vi "SERIAL_DecodeASCII.vi"(2 "navX Data":u8[](array[numeric]), 3 "Buffer":string) -> (0 "navX Data":u8[](array[numeric]), 1 "Valid?":bool)   [LabVIEW 2014, in "navX-MXP IMU.lvlib"]
uses:
  navX-MXP IMU.lvlib
  COMMON/TypeDefs/Value TypeDefs/navX Device Registers.ctl
  COMMON/TypeDefs/Value TypeDefs/navX NAVX_CAL_STATUS.ctl
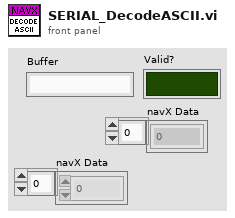
[diagram p1: front panel]
types:
  T1 = typedef "navX-MXP IMU.lvlib/navX Device Registers.ctl" = u8
  T2 = typedef "navX-MXP IMU.lvlib/navX NAVX_CAL_STATUS.ctl" = u8
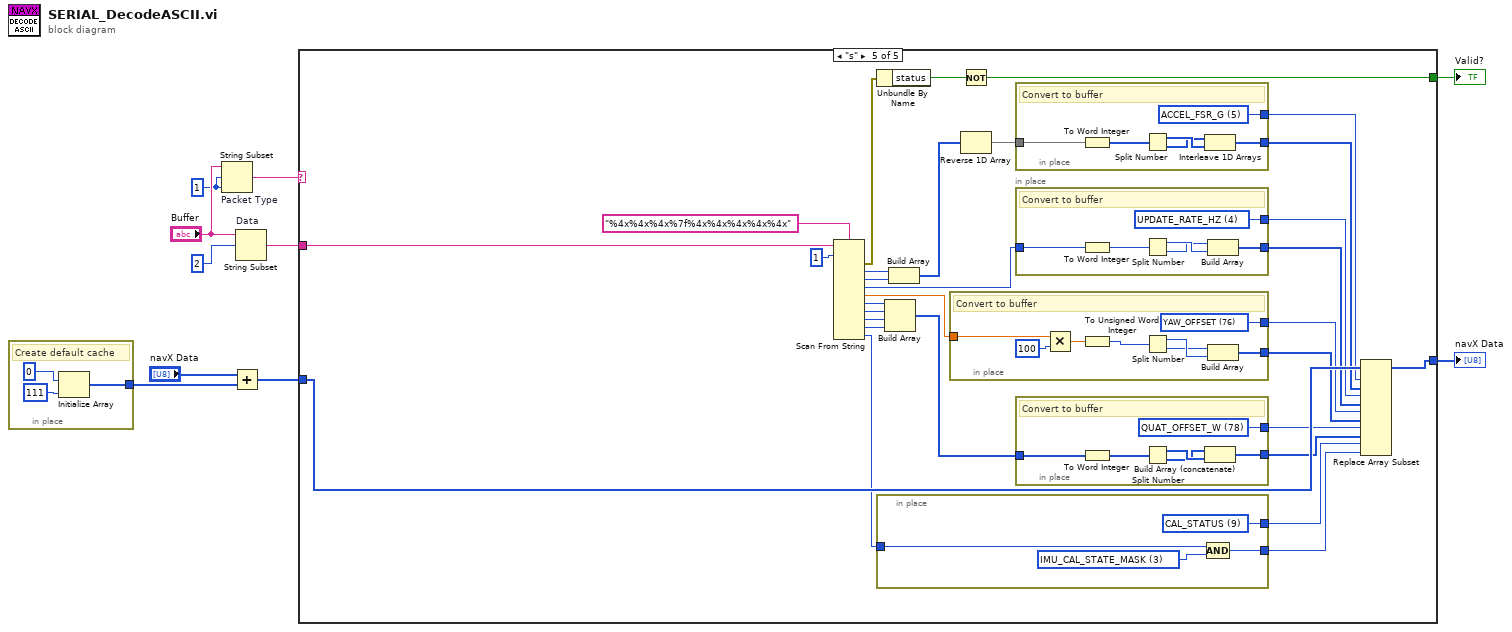
[diagram p0: block diagram]
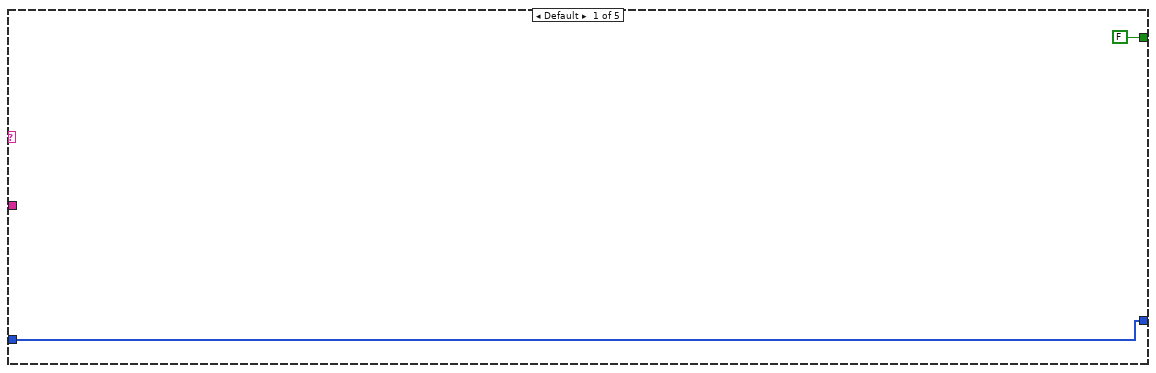
[diagram p2: hidden frame]
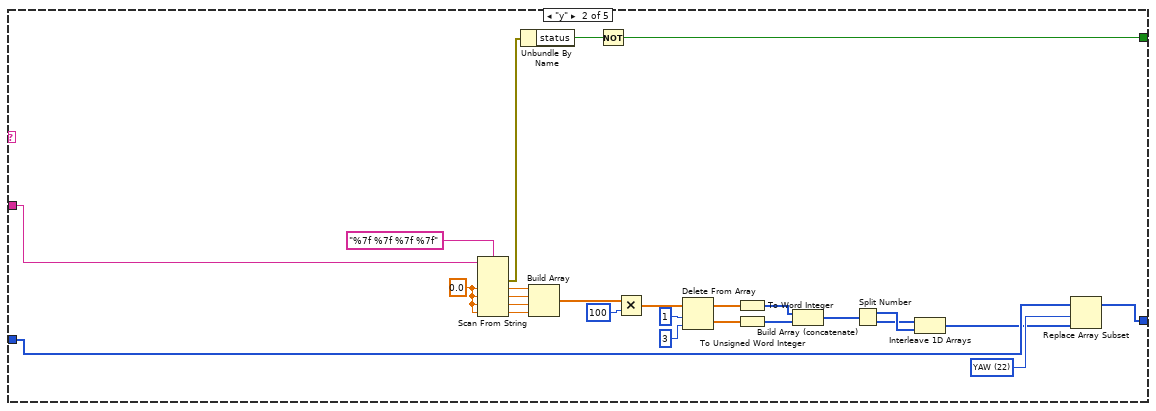
[diagram p3: hidden frame]
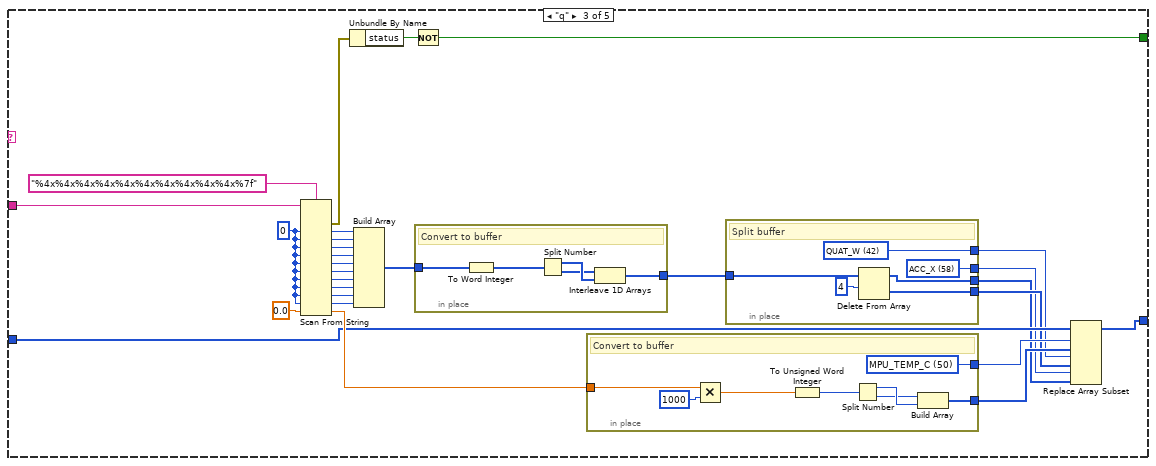
[diagram p4: hidden frame]
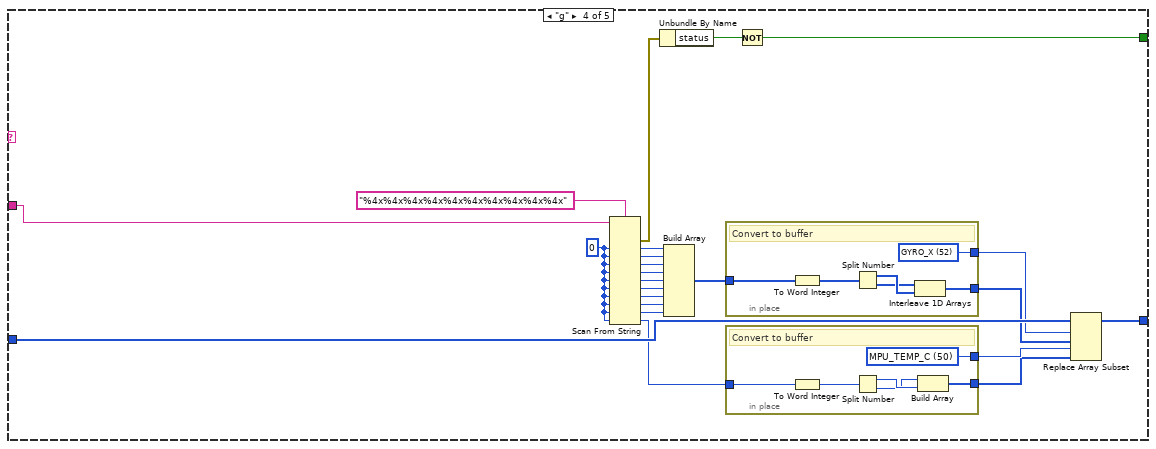
[diagram p5: hidden frame]
diagram:
  w8 = 1 ("offset (0)")
  n1 = in-place {
    in-place-border: [w11] -> w3
    # "Create default cache"
    n2 = Initialize Array(u8 0 ("Received Data"), u8 111 ("hex")) -> (w11:u8[])
  }
  n3 = String Subset "Packet Type"(string="Buffer", offset (0)=w8, length (rest)=w8) -> (substring=w7:string)
  n4 = Add(x="navX Data", y=w3) -> (x+y=w2:u8[])
  n5 = String Subset "Data"(string="Buffer", offset (0)=2) -> (substring=w1:string)  [unwired: 1 in]
  n6 = case shown="\"s\"" w7 {
    tunnel: w1 -> [_ w40 w65 w89 w124]
    tunnel: w2 -> [w15 w32 w50 w100 w147]
    tunnel: [w15 w30 w49 w97 w148] -> w6
    tunnel: [FALSE w16 w51 w94 w149] -> w5
    frame Default {
    }
    frame "y" {
      w31 = T1 22 items=["WHOAMI"=0, "HW_REV"=1, "FW_VER_MAJOR"=2, "FW_VER_MINOR"=3, "UPDATE_RATE_HZ"=4, "ACCEL_FSR_G"=5, "GYRO_FSR_DPS"=6, "OP_STATUS"=8, "CAL_STATUS"=9, "SELFTEST_STATUS"=10, "CAPABILITY_FLAGS_L"=11, "CAPABILITY_FLAGS_H"=12, "SENSOR_STATUS"=16, "TIMESTAMP"=18, "YAW"=22, "PITCH"=24, "ROLL"=26, "HEADING"=28, "FUSED_HEADING"=30, "ALTITUDE_I"=32, "ALTITUDE_D"=34, "LINERA_ACC_X"=36, "LINERA_ACC_Y"=38, "LINERA_ACC_Z"=40, "QUAT_W"=42, "QUAT_X"=44, "QUAT_Y"=46, "QUAT_Z"=48, "MPU_TEMP_C"=50, "GYRO_X"=52, "GYRO_Y"=54, "GYRO_Z"=56, "ACC_X"=58, "ACC_Y"=60, "ACC_Z"=62, "MAG_X"=64, "MAG_Y"=66, "MAG_Z"=68, "PRESSURE_I"=70, "PRESSURE_D"=72, "PRESSURE_TEMP"=74, "YAW_OFFSET"=76, "QUAT_OFFSET_W"=78, "QUAT_OFFSET_X"=80, "QUAT_OFFSET_Y"=82, "QUAT_OFFSET_Z"=84, "INTEGRATION_CONTROL"=86, "VELOCITY_X"=88, "VELOCITY_Y"=92, "VELOCITY_Z"=96, "DISPLACMENT_X"=100, "DISPLACMENT_Y"=104, "DISPLACEMENT_Z"=108] ("Device Register")
      w39 = 0.0 ("default value 1")
      n7 = Scan From String(format string="%7f %7f %7f %7f", input string=w40, default 1=w39, default 2=w39, default 3=w39, default 4=w39) -> (error out=w18:errorcluster, output 1=w38:dbl, output 2=w35:dbl, output 3=w36:dbl, output 4=w37:dbl)  [unwired: 2 in, 2 out]
      n8 = Unbundle By Name(w18) -> ("status"=w17:bool)
      n9 = Build Array(w38, w35, w36, w37) -> (w34:dbl[])
      n10 = Not(x=w17) -> (.not. x?=w16:bool)
      n11 = Multiply(x=w34, y=u16 100) -> (x*y=w20:dbl[])
      n12 = Delete From Array(array=w20, length=1, index=3) -> (deleted portion=w25:dbl[], array with subset deleted=w24:dbl[])
      n13 = To Word Integer(number=w24) -> (16bit integer=w23:i16[])
      n14 = To Unsigned Word Integer(number=w25) -> (unsigned 16bit integer=w22:u16[])
      n15 = Build Array (concatenate)(w23, w22) -> (w21:u16[])
      n16 = Split Number(x=w21) -> (hi(x)=w29:u8[], lo(x)=w28:u8[])
      n17 = Interleave 1D Arrays(w28, w29) -> (w19:u8[])
      n18 = Replace Array Subset(array=w32, new element=w19, index=w31) -> (w30:u8[])
    }
    frame "q" {
      w66 = u32 0 ("default value 1")
      n19 = Scan From String(format string="%4x%4x%4x%4x%4x%4x%4x%4x%4x%4x%7f", input string=w65, default 1=w66, default 2=w66, default 3=w66, default 4=w66, default 5=w66, default 6=w66, default 7=w66, default 8=w66, default 9=w66, default 10=w66, default 11=0.0 ("default value 11")) -> (error out=w67:errorcluster, output 1=w62:u32, output 2=w61:u32, output 3=w60:u32, output 4=w59:u32, output 5=w58:u32, output 6=w57:u32, output 7=w56:u32, output 8=w55:u32, output 9=w54:u32, output 10=w53:u32, output 11=w52:dbl)  [unwired: 2 in, 2 out]
      n20 = Unbundle By Name(w67) -> ("status"=w68:bool)
      n21 = Build Array(w62, w61, w60, w59, w58, w57, w56, w55, w54, w53) -> (w63:u32[])
      n22 = Not(x=w68) -> (.not. x?=w51:bool)
      n23 = in-place {
        in-place-border: w63 -> [w88]
        in-place-border: [w84] -> w46
        # "Convert to buffer"
        n24 = To Word Integer(number=w88) -> (16bit integer=w85:i16[])
        n25 = Split Number(x=w85) -> (hi(x)=w87:u8[], lo(x)=w86:u8[])
        n26 = Interleave 1D Arrays(w86, w87) -> (w84:u8[])
      }
      n27 = in-place {
        in-place-border: w52 -> [w80]
        in-place-border: [w77] -> w47
        in-place-border: [w76] -> w48
        w76 = T1 50 items=["WHOAMI"=0, "HW_REV"=1, "FW_VER_MAJOR"=2, "FW_VER_MINOR"=3, "UPDATE_RATE_HZ"=4, "ACCEL_FSR_G"=5, "GYRO_FSR_DPS"=6, "OP_STATUS"=8, "CAL_STATUS"=9, "SELFTEST_STATUS"=10, "CAPABILITY_FLAGS_L"=11, "CAPABILITY_FLAGS_H"=12, "SENSOR_STATUS"=16, "TIMESTAMP"=18, "YAW"=22, "PITCH"=24, "ROLL"=26, "HEADING"=28, "FUSED_HEADING"=30, "ALTITUDE_I"=32, "ALTITUDE_D"=34, "LINERA_ACC_X"=36, "LINERA_ACC_Y"=38, "LINERA_ACC_Z"=40, "QUAT_W"=42, "QUAT_X"=44, "QUAT_Y"=46, "QUAT_Z"=48, "MPU_TEMP_C"=50, "GYRO_X"=52, "GYRO_Y"=54, "GYRO_Z"=56, "ACC_X"=58, "ACC_Y"=60, "ACC_Z"=62, "MAG_X"=64, "MAG_Y"=66, "MAG_Z"=68, "PRESSURE_I"=70, "PRESSURE_D"=72, "PRESSURE_TEMP"=74, "YAW_OFFSET"=76, "QUAT_OFFSET_W"=78, "QUAT_OFFSET_X"=80, "QUAT_OFFSET_Y"=82, "QUAT_OFFSET_Z"=84, "INTEGRATION_CONTROL"=86, "VELOCITY_X"=88, "VELOCITY_Y"=92, "VELOCITY_Z"=96, "DISPLACMENT_X"=100, "DISPLACMENT_Y"=104, "DISPLACEMENT_Z"=108] ("Device Register")
        # "Convert to buffer"
        n28 = Multiply(x=w80, y=u16 1000) -> (x*y=w79:dbl)
        n29 = To Unsigned Word Integer(number=w79) -> (unsigned 16bit integer=w78:u16)
        n30 = Split Number(x=w78) -> (hi(x)=w82:u8, lo(x)=w81:u8)
        n31 = Build Array(w81, w82) -> (w77:u8[])
      }
      n32 = in-place {
        in-place-border: w46 -> [w75]
        in-place-border: [w73] -> w45
        in-place-border: [w72] -> w44
        in-place-border: [w71] -> w43
        in-place-border: [w70] -> w42
        w70 = T1 58 items=["WHOAMI"=0, "HW_REV"=1, "FW_VER_MAJOR"=2, "FW_VER_MINOR"=3, "UPDATE_RATE_HZ"=4, "ACCEL_FSR_G"=5, "GYRO_FSR_DPS"=6, "OP_STATUS"=8, "CAL_STATUS"=9, "SELFTEST_STATUS"=10, "CAPABILITY_FLAGS_L"=11, "CAPABILITY_FLAGS_H"=12, "SENSOR_STATUS"=16, "TIMESTAMP"=18, "YAW"=22, "PITCH"=24, "ROLL"=26, "HEADING"=28, "FUSED_HEADING"=30, "ALTITUDE_I"=32, "ALTITUDE_D"=34, "LINERA_ACC_X"=36, "LINERA_ACC_Y"=38, "LINERA_ACC_Z"=40, "QUAT_W"=42, "QUAT_X"=44, "QUAT_Y"=46, "QUAT_Z"=48, "MPU_TEMP_C"=50, "GYRO_X"=52, "GYRO_Y"=54, "GYRO_Z"=56, "ACC_X"=58, "ACC_Y"=60, "ACC_Z"=62, "MAG_X"=64, "MAG_Y"=66, "MAG_Z"=68, "PRESSURE_I"=70, "PRESSURE_D"=72, "PRESSURE_TEMP"=74, "YAW_OFFSET"=76, "QUAT_OFFSET_W"=78, "QUAT_OFFSET_X"=80, "QUAT_OFFSET_Y"=82, "QUAT_OFFSET_Z"=84, "INTEGRATION_CONTROL"=86, "VELOCITY_X"=88, "VELOCITY_Y"=92, "VELOCITY_Z"=96, "DISPLACMENT_X"=100, "DISPLACMENT_Y"=104, "DISPLACEMENT_Z"=108] ("Device Register")
        w72 = T1 42 items=["WHOAMI"=0, "HW_REV"=1, "FW_VER_MAJOR"=2, "FW_VER_MINOR"=3, "UPDATE_RATE_HZ"=4, "ACCEL_FSR_G"=5, "GYRO_FSR_DPS"=6, "OP_STATUS"=8, "CAL_STATUS"=9, "SELFTEST_STATUS"=10, "CAPABILITY_FLAGS_L"=11, "CAPABILITY_FLAGS_H"=12, "SENSOR_STATUS"=16, "TIMESTAMP"=18, "YAW"=22, "PITCH"=24, "ROLL"=26, "HEADING"=28, "FUSED_HEADING"=30, "ALTITUDE_I"=32, "ALTITUDE_D"=34, "LINERA_ACC_X"=36, "LINERA_ACC_Y"=38, "LINERA_ACC_Z"=40, "QUAT_W"=42, "QUAT_X"=44, "QUAT_Y"=46, "QUAT_Z"=48, "MPU_TEMP_C"=50, "GYRO_X"=52, "GYRO_Y"=54, "GYRO_Z"=56, "ACC_X"=58, "ACC_Y"=60, "ACC_Z"=62, "MAG_X"=64, "MAG_Y"=66, "MAG_Z"=68, "PRESSURE_I"=70, "PRESSURE_D"=72, "PRESSURE_TEMP"=74, "YAW_OFFSET"=76, "QUAT_OFFSET_W"=78, "QUAT_OFFSET_X"=80, "QUAT_OFFSET_Y"=82, "QUAT_OFFSET_Z"=84, "INTEGRATION_CONTROL"=86, "VELOCITY_X"=88, "VELOCITY_Y"=92, "VELOCITY_Z"=96, "DISPLACMENT_X"=100, "DISPLACMENT_Y"=104, "DISPLACEMENT_Z"=108] ("Device Register")
        # "Split buffer"
        n33 = Delete From Array(array=w75, length=4) -> (deleted portion=w73:u8[], array with subset deleted=w71:u8[])  [unwired: 1 in]
      }
      n34 = Replace Array Subset(array=w50, new element #1=w47, index #1=w48, new element #2=w45, index #2=w44, new element #3=w43, index #3=w42) -> (w49:u8[])
    }
    frame "g" {
      w90 = u32 0 ("default value 1")
      n35 = Scan From String(format string="%4x%4x%4x%4x%4x%4x%4x%4x%4x%4x", input string=w89, default 1=w90, default 2=w90, default 3=w90, default 4=w90, default 5=w90, default 6=w90, default 7=w90, default 8=w90, default 9=w90, default 10=w90) -> (error out=w95:errorcluster, output 1=w110:u32, output 2=w109:u32, output 3=w108:u32, output 4=w106:u32, output 5=w105:u32, output 6=w104:u32, output 7=w103:u32, output 8=w102:u32, output 9=w101:u32, output 10=w93:u32)  [unwired: 2 in, 2 out]
      n36 = Unbundle By Name(w95) -> ("status"=w96:bool)
      n37 = Build Array(w110, w109, w108, w106, w105, w104, w103, w102, w101) -> (w107:u32[])
      n38 = in-place {
        in-place-border: w107 -> [w123]
        in-place-border: [w119] -> w99
        in-place-border: [w118] -> w98
        w118 = T1 52 items=["WHOAMI"=0, "HW_REV"=1, "FW_VER_MAJOR"=2, "FW_VER_MINOR"=3, "UPDATE_RATE_HZ"=4, "ACCEL_FSR_G"=5, "GYRO_FSR_DPS"=6, "OP_STATUS"=8, "CAL_STATUS"=9, "SELFTEST_STATUS"=10, "CAPABILITY_FLAGS_L"=11, "CAPABILITY_FLAGS_H"=12, "SENSOR_STATUS"=16, "TIMESTAMP"=18, "YAW"=22, "PITCH"=24, "ROLL"=26, "HEADING"=28, "FUSED_HEADING"=30, "ALTITUDE_I"=32, "ALTITUDE_D"=34, "LINERA_ACC_X"=36, "LINERA_ACC_Y"=38, "LINERA_ACC_Z"=40, "QUAT_W"=42, "QUAT_X"=44, "QUAT_Y"=46, "QUAT_Z"=48, "MPU_TEMP_C"=50, "GYRO_X"=52, "GYRO_Y"=54, "GYRO_Z"=56, "ACC_X"=58, "ACC_Y"=60, "ACC_Z"=62, "MAG_X"=64, "MAG_Y"=66, "MAG_Z"=68, "PRESSURE_I"=70, "PRESSURE_D"=72, "PRESSURE_TEMP"=74, "YAW_OFFSET"=76, "QUAT_OFFSET_W"=78, "QUAT_OFFSET_X"=80, "QUAT_OFFSET_Y"=82, "QUAT_OFFSET_Z"=84, "INTEGRATION_CONTROL"=86, "VELOCITY_X"=88, "VELOCITY_Y"=92, "VELOCITY_Z"=96, "DISPLACMENT_X"=100, "DISPLACMENT_Y"=104, "DISPLACEMENT_Z"=108] ("Device Register")
        # "Convert to buffer"
        n39 = To Word Integer(number=w123) -> (16bit integer=w120:i16[])
        n40 = Split Number(x=w120) -> (hi(x)=w122:u8[], lo(x)=w121:u8[])
        n41 = Interleave 1D Arrays(w121, w122) -> (w119:u8[])
      }
      n42 = in-place {
        in-place-border: w93 -> [w113]
        in-place-border: [w115] -> w92
        in-place-border: [w114] -> w91
        w115 = T1 50 items=["WHOAMI"=0, "HW_REV"=1, "FW_VER_MAJOR"=2, "FW_VER_MINOR"=3, "UPDATE_RATE_HZ"=4, "ACCEL_FSR_G"=5, "GYRO_FSR_DPS"=6, "OP_STATUS"=8, "CAL_STATUS"=9, "SELFTEST_STATUS"=10, "CAPABILITY_FLAGS_L"=11, "CAPABILITY_FLAGS_H"=12, "SENSOR_STATUS"=16, "TIMESTAMP"=18, "YAW"=22, "PITCH"=24, "ROLL"=26, "HEADING"=28, "FUSED_HEADING"=30, "ALTITUDE_I"=32, "ALTITUDE_D"=34, "LINERA_ACC_X"=36, "LINERA_ACC_Y"=38, "LINERA_ACC_Z"=40, "QUAT_W"=42, "QUAT_X"=44, "QUAT_Y"=46, "QUAT_Z"=48, "MPU_TEMP_C"=50, "GYRO_X"=52, "GYRO_Y"=54, "GYRO_Z"=56, "ACC_X"=58, "ACC_Y"=60, "ACC_Z"=62, "MAG_X"=64, "MAG_Y"=66, "MAG_Z"=68, "PRESSURE_I"=70, "PRESSURE_D"=72, "PRESSURE_TEMP"=74, "YAW_OFFSET"=76, "QUAT_OFFSET_W"=78, "QUAT_OFFSET_X"=80, "QUAT_OFFSET_Y"=82, "QUAT_OFFSET_Z"=84, "INTEGRATION_CONTROL"=86, "VELOCITY_X"=88, "VELOCITY_Y"=92, "VELOCITY_Z"=96, "DISPLACMENT_X"=100, "DISPLACMENT_Y"=104, "DISPLACEMENT_Z"=108] ("Device Register")
        # "Convert to buffer"
        n43 = To Word Integer(number=w113) -> (16bit integer=w112:i16)
        n44 = Split Number(x=w112) -> (hi(x)=w117:u8, lo(x)=w116:u8)
        n45 = Build Array(w116, w117) -> (w114:u8[])
      }
      n46 = Not(x=w96) -> (.not. x?=w94:bool)
      n47 = Replace Array Subset(array=w100, new element #1=w99, index #1=w98, new element #2=w91, index #2=w92) -> (w97:u8[])
    }
    frame "s" {
      n48 = Scan From String(format string="%4x%4x%4x%7f%4x%4x%4x%4x%4x", input string=w124, initial scan location=u32 1) -> (error out=w150:errorcluster, output 1=w146:u32, output 2=w145:u32, output 3=w140:u32, output 4=w137:dbl, output 5=w134:u32, output 6=w133:u32, output 7=w132:u32, output 8=w131:u32, output 9=w127:u32)  [unwired: 10 in, 2 out]
      n49 = Unbundle By Name(w150) -> ("status"=w151:bool)
      n50 = in-place {
        in-place-border: w127 -> [w156]
        in-place-border: [w155] -> w126
        in-place-border: [w154] -> w125
        w155 = T1 9 items=["WHOAMI"=0, "HW_REV"=1, "FW_VER_MAJOR"=2, "FW_VER_MINOR"=3, "UPDATE_RATE_HZ"=4, "ACCEL_FSR_G"=5, "GYRO_FSR_DPS"=6, "OP_STATUS"=8, "CAL_STATUS"=9, "SELFTEST_STATUS"=10, "CAPABILITY_FLAGS_L"=11, "CAPABILITY_FLAGS_H"=12, "SENSOR_STATUS"=16, "TIMESTAMP"=18, "YAW"=22, "PITCH"=24, "ROLL"=26, "HEADING"=28, "FUSED_HEADING"=30, "ALTITUDE_I"=32, "ALTITUDE_D"=34, "LINERA_ACC_X"=36, "LINERA_ACC_Y"=38, "LINERA_ACC_Z"=40, "QUAT_W"=42, "QUAT_X"=44, "QUAT_Y"=46, "QUAT_Z"=48, "MPU_TEMP_C"=50, "GYRO_X"=52, "GYRO_Y"=54, "GYRO_Z"=56, "ACC_X"=58, "ACC_Y"=60, "ACC_Z"=62, "MAG_X"=64, "MAG_Y"=66, "MAG_Z"=68, "PRESSURE_I"=70, "PRESSURE_D"=72, "PRESSURE_TEMP"=74, "YAW_OFFSET"=76, "QUAT_OFFSET_W"=78, "QUAT_OFFSET_X"=80, "QUAT_OFFSET_Y"=82, "QUAT_OFFSET_Z"=84, "INTEGRATION_CONTROL"=86, "VELOCITY_X"=88, "VELOCITY_Y"=92, "VELOCITY_Z"=96, "DISPLACMENT_X"=100, "DISPLACMENT_Y"=104, "DISPLACEMENT_Z"=108] ("Device Register")
        w157 = T2 3 items=["IMU_CAL_STATE_MASK"=3, "IMU_CAL_INPROGRESS"=0, "IMU_CAL_ACCUMULATE"=1, "IMU_CAL_COMPLETE"=2, "MAG_CAL_COMPLETE"=4, "BARO_CAL_COMPLETE"=8] ("NAVX_CAL_STATUS")
        n51 = Compound Arithmetic op=AND(w156, w157) -> (w154:u32)
      }
      n52 = Build Array(w134, w133, w132, w131) -> (w130:u32[])
      n53 = Build Array(w146, w145) -> (w144:u32[])
      n54 = in-place {
        in-place-border: w137 -> [w168]
        in-place-border: [w165] -> w135
        in-place-border: [w164] -> w136
        w164 = T1 76 items=["WHOAMI"=0, "HW_REV"=1, "FW_VER_MAJOR"=2, "FW_VER_MINOR"=3, "UPDATE_RATE_HZ"=4, "ACCEL_FSR_G"=5, "GYRO_FSR_DPS"=6, "OP_STATUS"=8, "CAL_STATUS"=9, "SELFTEST_STATUS"=10, "CAPABILITY_FLAGS_L"=11, "CAPABILITY_FLAGS_H"=12, "SENSOR_STATUS"=16, "TIMESTAMP"=18, "YAW"=22, "PITCH"=24, "ROLL"=26, "HEADING"=28, "FUSED_HEADING"=30, "ALTITUDE_I"=32, "ALTITUDE_D"=34, "LINERA_ACC_X"=36, "LINERA_ACC_Y"=38, "LINERA_ACC_Z"=40, "QUAT_W"=42, "QUAT_X"=44, "QUAT_Y"=46, "QUAT_Z"=48, "MPU_TEMP_C"=50, "GYRO_X"=52, "GYRO_Y"=54, "GYRO_Z"=56, "ACC_X"=58, "ACC_Y"=60, "ACC_Z"=62, "MAG_X"=64, "MAG_Y"=66, "MAG_Z"=68, "PRESSURE_I"=70, "PRESSURE_D"=72, "PRESSURE_TEMP"=74, "YAW_OFFSET"=76, "QUAT_OFFSET_W"=78, "QUAT_OFFSET_X"=80, "QUAT_OFFSET_Y"=82, "QUAT_OFFSET_Z"=84, "INTEGRATION_CONTROL"=86, "VELOCITY_X"=88, "VELOCITY_Y"=92, "VELOCITY_Z"=96, "DISPLACMENT_X"=100, "DISPLACMENT_Y"=104, "DISPLACEMENT_Z"=108] ("Device Register")
        # "Convert to buffer"
        n55 = Multiply(x=w168, y=u16 100) -> (x*y=w167:dbl)
        n56 = To Unsigned Word Integer(number=w167) -> (unsigned 16bit integer=w166:u16)
        n57 = Split Number(x=w166) -> (hi(x)=w170:u8, lo(x)=w169:u8)
        n58 = Build Array(w169, w170) -> (w165:u8[])
      }
      n59 = Not(x=w151) -> (.not. x?=w149:bool)
      n60 = Reverse 1D Array(array=w144) -> (reversed array=w143:u32[])
      n61 = in-place {
        in-place-border: w143 -> [w183]
        in-place-border: [w179] -> w141
        in-place-border: [w178] -> w142
        w178 = T1 5 items=["WHOAMI"=0, "HW_REV"=1, "FW_VER_MAJOR"=2, "FW_VER_MINOR"=3, "UPDATE_RATE_HZ"=4, "ACCEL_FSR_G"=5, "GYRO_FSR_DPS"=6, "OP_STATUS"=8, "CAL_STATUS"=9, "SELFTEST_STATUS"=10, "CAPABILITY_FLAGS_L"=11, "CAPABILITY_FLAGS_H"=12, "SENSOR_STATUS"=16, "TIMESTAMP"=18, "YAW"=22, "PITCH"=24, "ROLL"=26, "HEADING"=28, "FUSED_HEADING"=30, "ALTITUDE_I"=32, "ALTITUDE_D"=34, "LINERA_ACC_X"=36, "LINERA_ACC_Y"=38, "LINERA_ACC_Z"=40, "QUAT_W"=42, "QUAT_X"=44, "QUAT_Y"=46, "QUAT_Z"=48, "MPU_TEMP_C"=50, "GYRO_X"=52, "GYRO_Y"=54, "GYRO_Z"=56, "ACC_X"=58, "ACC_Y"=60, "ACC_Z"=62, "MAG_X"=64, "MAG_Y"=66, "MAG_Z"=68, "PRESSURE_I"=70, "PRESSURE_D"=72, "PRESSURE_TEMP"=74, "YAW_OFFSET"=76, "QUAT_OFFSET_W"=78, "QUAT_OFFSET_X"=80, "QUAT_OFFSET_Y"=82, "QUAT_OFFSET_Z"=84, "INTEGRATION_CONTROL"=86, "VELOCITY_X"=88, "VELOCITY_Y"=92, "VELOCITY_Z"=96, "DISPLACMENT_X"=100, "DISPLACMENT_Y"=104, "DISPLACEMENT_Z"=108] ("Device Register")
        # "Convert to buffer"
        n62 = To Word Integer(number=w183) -> (16bit integer=w180:i16[])
        n63 = Split Number(x=w180) -> (hi(x)=w182:u8[], lo(x)=w181:u8[])
        n64 = Interleave 1D Arrays(w181, w182) -> (w179:u8[])
      }
      n65 = in-place {
        in-place-border: w140 -> [w177]
        in-place-border: [w173] -> w138
        in-place-border: [w172] -> w139
        w172 = T1 4 items=["WHOAMI"=0, "HW_REV"=1, "FW_VER_MAJOR"=2, "FW_VER_MINOR"=3, "UPDATE_RATE_HZ"=4, "ACCEL_FSR_G"=5, "GYRO_FSR_DPS"=6, "OP_STATUS"=8, "CAL_STATUS"=9, "SELFTEST_STATUS"=10, "CAPABILITY_FLAGS_L"=11, "CAPABILITY_FLAGS_H"=12, "SENSOR_STATUS"=16, "TIMESTAMP"=18, "YAW"=22, "PITCH"=24, "ROLL"=26, "HEADING"=28, "FUSED_HEADING"=30, "ALTITUDE_I"=32, "ALTITUDE_D"=34, "LINERA_ACC_X"=36, "LINERA_ACC_Y"=38, "LINERA_ACC_Z"=40, "QUAT_W"=42, "QUAT_X"=44, "QUAT_Y"=46, "QUAT_Z"=48, "MPU_TEMP_C"=50, "GYRO_X"=52, "GYRO_Y"=54, "GYRO_Z"=56, "ACC_X"=58, "ACC_Y"=60, "ACC_Z"=62, "MAG_X"=64, "MAG_Y"=66, "MAG_Z"=68, "PRESSURE_I"=70, "PRESSURE_D"=72, "PRESSURE_TEMP"=74, "YAW_OFFSET"=76, "QUAT_OFFSET_W"=78, "QUAT_OFFSET_X"=80, "QUAT_OFFSET_Y"=82, "QUAT_OFFSET_Z"=84, "INTEGRATION_CONTROL"=86, "VELOCITY_X"=88, "VELOCITY_Y"=92, "VELOCITY_Z"=96, "DISPLACMENT_X"=100, "DISPLACMENT_Y"=104, "DISPLACEMENT_Z"=108] ("Device Register")
        # "Convert to buffer"
        n66 = To Word Integer(number=w177) -> (16bit integer=w174:i16)
        n67 = Split Number(x=w174) -> (hi(x)=w176:u8, lo(x)=w175:u8)
        n68 = Build Array(w175, w176) -> (w173:u8[])
      }
      n69 = in-place {
        in-place-border: w130 -> [w163]
        in-place-border: [w159] -> w128
        in-place-border: [w158] -> w129
        w158 = T1 78 items=["WHOAMI"=0, "HW_REV"=1, "FW_VER_MAJOR"=2, "FW_VER_MINOR"=3, "UPDATE_RATE_HZ"=4, "ACCEL_FSR_G"=5, "GYRO_FSR_DPS"=6, "OP_STATUS"=8, "CAL_STATUS"=9, "SELFTEST_STATUS"=10, "CAPABILITY_FLAGS_L"=11, "CAPABILITY_FLAGS_H"=12, "SENSOR_STATUS"=16, "TIMESTAMP"=18, "YAW"=22, "PITCH"=24, "ROLL"=26, "HEADING"=28, "FUSED_HEADING"=30, "ALTITUDE_I"=32, "ALTITUDE_D"=34, "LINERA_ACC_X"=36, "LINERA_ACC_Y"=38, "LINERA_ACC_Z"=40, "QUAT_W"=42, "QUAT_X"=44, "QUAT_Y"=46, "QUAT_Z"=48, "MPU_TEMP_C"=50, "GYRO_X"=52, "GYRO_Y"=54, "GYRO_Z"=56, "ACC_X"=58, "ACC_Y"=60, "ACC_Z"=62, "MAG_X"=64, "MAG_Y"=66, "MAG_Z"=68, "PRESSURE_I"=70, "PRESSURE_D"=72, "PRESSURE_TEMP"=74, "YAW_OFFSET"=76, "QUAT_OFFSET_W"=78, "QUAT_OFFSET_X"=80, "QUAT_OFFSET_Y"=82, "QUAT_OFFSET_Z"=84, "INTEGRATION_CONTROL"=86, "VELOCITY_X"=88, "VELOCITY_Y"=92, "VELOCITY_Z"=96, "DISPLACMENT_X"=100, "DISPLACMENT_Y"=104, "DISPLACEMENT_Z"=108] ("Device Register")
        # "Convert to buffer"
        n70 = To Word Integer(number=w163) -> (16bit integer=w160:i16[])
        n71 = Split Number(x=w160) -> (hi(x)=w162:u8[], lo(x)=w161:u8[])
        n72 = Build Array (concatenate)(w161, w162) -> (w159:u8[])
      }
      n73 = Replace Array Subset(array=w147, new element #1=w141, index #1=w142, new element #2=w138, index #2=w139, new element #3=w135, index #3=w136, new element #4=w128, index #4=w129, new element #5=w125, index #5=w126) -> (w148:u8[])
    }
  }
  "Valid?" <- w5
  "navX Data" <- w6
